vi "pump_server.vi"(10 "pump load":bool, 11 "Serial Port in":refnum<visa-resource-name>) -> ()   [LabVIEW 2020]
uses:
  status/stop software.vi
  status/emergency stop.vi
panel:
  in  "error in (no error)":errorcluster
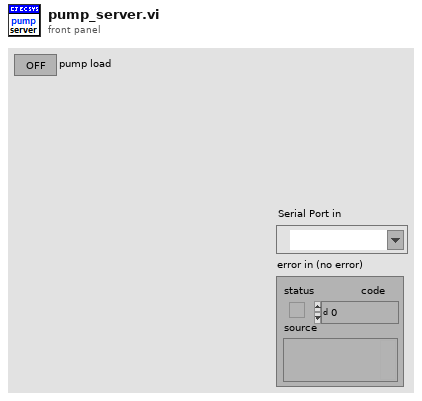
[diagram p1: front panel]
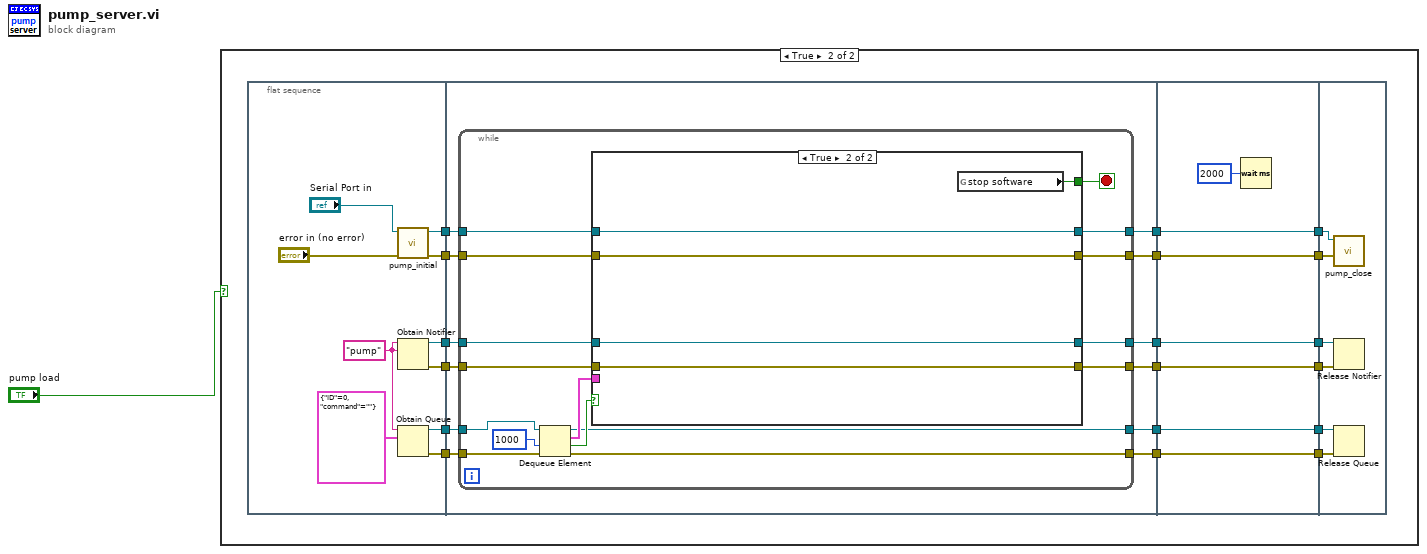
[diagram p0: block diagram]
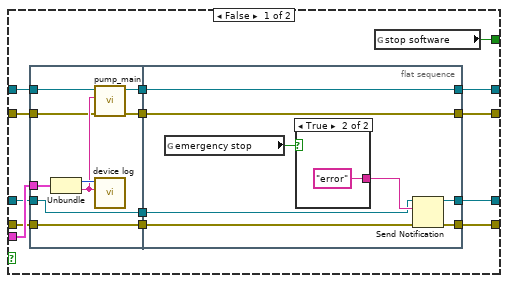
[diagram p3: hidden frame]
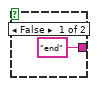
[diagram p4: hidden frame]
diagram:
  n1 = case shown="True" "pump load" {
    frame False {
    }
    frame True {
      n2 = flat-sequence {
        tunnel: [w29] -> w19
        tunnel: [w28] -> w18
        tunnel: [w27] -> w17
        tunnel: [w26] -> w16
        tunnel: [w20] -> w15
        tunnel: [w21] -> w14
        tunnel: w19 -> [w41]
        tunnel: w18 -> [w40]
        tunnel: w17 -> [w39]
        tunnel: w16 -> [w38]
        tunnel: [w37] -> w13
        tunnel: [w36] -> w12
        tunnel: [w35] -> w11
        tunnel: [w34] -> w10
        tunnel: w15 -> [w33]
        tunnel: w14 -> [w32]
        tunnel: [w31] -> w9
        tunnel: [w30] -> w8
        tunnel: w13 -> [w102]
        tunnel: [w102] -> w7
        tunnel: w12 -> [w101]
        tunnel: [w101] -> w6
        tunnel: w11 -> [w100]
        tunnel: [w100] -> w5
        tunnel: w10 -> [w99]
        tunnel: [w99] -> w4
        tunnel: w9 -> [w98]
        tunnel: [w98] -> w3
        tunnel: w8 -> [w97]
        tunnel: [w97] -> w2
        tunnel: w7 -> [w108]
        tunnel: w6 -> [w107]
        tunnel: w5 -> [w106]
        tunnel: w4 -> [w105]
        tunnel: w3 -> [w104]
        tunnel: w2 -> [w103]
        frame #0 {
          w25 = "pump" ("name (unnamed)")
          n3 = call "pump_initial.vi"("error in (no error)"="error in (no error)", "Serial Port in"="Serial Port in") -> ("error out"=w21:errorcluster, "Serial Port out"=w20:refnum<visa-resource-name>)  [unwired: 8 in]
          n4 = Obtain Notifier(name (unnamed)=w25, notification data type=w25) -> (notifier out=w27:refnum<notifier>, error out=w26:errorcluster)  [unwired: 2 in, 1 out]
          n5 = Obtain Queue(name (unnamed)=w25, element data type=cluster{"ID":i32, "command":string} {"ID"=0, "command"=""} ("参数")) -> (queue out=w29:refnum<queue>, error out=w28:errorcluster)  [unwired: 3 in, 1 out]
        }
        frame #1 {
          n6 = while {
            tunnel: w41 -> [w56]
            tunnel: w40 -> [w55]
            tunnel: w39 -> [w51]
            tunnel: w38 -> [w50]
            tunnel: [w49] -> w37
            tunnel: [w48] -> w36
            tunnel: [w47] -> w35
            tunnel: [w46] -> w34
            tunnel: w33 -> [w45]
            tunnel: w32 -> [w44]
            tunnel: [w43] -> w31
            tunnel: [w42] -> w30
            stop <- w53 stop-if-true
            n7 = Dequeue Element(queue=w56, timeout in ms (-1)=1000, error in (no error)=w55) -> (queue out=w47:refnum<queue>, element=w52:cluster{"ID":i32, "command":string}, timed out?=w54:bool, error out=w46:errorcluster)
            n8 = case shown="True" w54 {
              tunnel: [w66 w93] -> w53
              tunnel: w52 -> [w69 _]
              tunnel: w51 -> [w68 w95]
              tunnel: w50 -> [w67 w94]
              tunnel: [w71 w95] -> w49
              tunnel: [w70 w94] -> w48
              tunnel: w45 -> [w62 w92]
              tunnel: w44 -> [w61 w91]
              tunnel: [w60 w92] -> w43
              tunnel: [w58 w91] -> w42
              frame False {
                n9 = flat-sequence {
                  tunnel: w69 -> [w78]
                  tunnel: w68 -> [w79]
                  tunnel: w67 -> [w80]
                  tunnel: [w80] -> w65
                  tunnel: [w79] -> w64
                  tunnel: [w75] -> w63
                  tunnel: w62 -> [w74]
                  tunnel: w61 -> [w73]
                  tunnel: [w72] -> w59
                  tunnel: [w87] -> w71
                  tunnel: [w86] -> w70
                  tunnel: w65 -> [w85]
                  tunnel: w64 -> [w83]
                  tunnel: w63 -> [w82]
                  tunnel: [w82] -> w60
                  tunnel: w59 -> [w81]
                  tunnel: [w81] -> w58
                  frame #0 {
                    n10 = Unbundle(w78) -> ("ID"=w77:i32, "command"=w76:string)
                    n11 = call "pump_main.vi"("error in (no error)"=w73, "input string"=w76, "VISA resource name"=w74) -> ("error out"=w72:errorcluster, "VISA resource name out"=w75:refnum<visa-resource-name>)  [unwired: 7 in]
                    n12 = call "device log.vi"("new element/subarray"=w76, "worker ID"=w77) -> ()  [unwired: 10 in]
                  }
                  frame #1 {
                    n13 = global read "emergency stop.vi" "emergency stop"() -> (w84:bool)
                    n14 = case shown="True" w84 {
                      tunnel: ["end" ("notification") "error" ("notification")] -> w88
                      frame False {
                      }
                      frame True {
                      }
                    }
                    n15 = Send Notification(notification=w88, notifier=w83, error in (no error)=w85) -> (notifier out=w87:refnum<notifier>, error out=w86:errorcluster)
                  }
                }
                n16 = global read "stop software.vi" "stop software"() -> (w66:bool)
              }
              frame True {
                n17 = global read "stop software.vi" "stop software"() -> (w93:bool)
              }
            }
          }
        }
        frame #2 {
          n18 = Wait (ms)(milliseconds to wait=u32 2000) -> ()  [unwired: 1 out]
        }
        frame #3 {
          n19 = call "pump_close.vi"("error in (no error)"=w103, "VISA resource name"=w104) -> ()  [unwired: 9 in, 1 out]
          n20 = Release Notifier(notifier=w108, error in (no error)=w107) -> ()  [unwired: 1 in, 3 out]
          n21 = Release Queue(queue=w106, error in (no error)=w105) -> ()  [unwired: 1 in, 3 out]
        }
      }
    }
  }
